vi "APC_PC_VariableMapping.vi"(3 "Index of array for 9056":i32[](array[numeric]), 4 "Index of array for 9049":i32[](array[numeric]), 5 "9056 IO":dbl[](array[numeric])=[0.0, 0.0, 0.0, 0.0, 0.0, 0.0, 0.0, 0.0, 0.0, 0.0, 0.0, 0.0, 0.0, 0.0, 0.0, 0.0, 0.0, 0.0, 0.0, 0.0, 0.0, 0.0, 0.0, 0.0, 0.0, 0.0, 0.0, 0.0, 0.0, 0.0, 0.0, 0.0, 0.0, 0.0, 0.0, 0.0, 0.0, 0.0, 0.0, 0.0, 0.0, 0.0, 0.0, 0.0, 0.0, 0.0, 0.0, 0.0, 0.0, 0.0], 6 "9049_CycleAveragedVariables":dbl[](array[numeric])=[5117258.0, 0.0, 0.0, 63.0, 1.0, 0.0, 0.0, 63.0, 94.902099609375, 1330.6719970703125, 0.00740314572500006, 0.028547040286386775, -1.6502519931731375e-05, 3.4809370619042162e-06, -1.939751072415059e-05, 0.04488519353144763, -3.310092996518957e-05, 1.9858346940817464e-05, -6.236978827880622e-06, 2.0827911733821188e-05, 9.443311193381779e-06, 0.006132818026759225, -2.7311908507416236e-05, 1.3270106306105403e-05, 0.028879043555142453, 0.028737060332811204, 0.028901641330023153, 22.045927206155966, 0.028741237014095793, 0.028786486597229075, 3.2774645046213114e-05, 1.6115711762159127e-05, 2.1821578936881718e-05, 0.03357141441039388, 2.0112356950239074e-05, 1.675670602532866e-05, 0.0006356573050482991, 0.0006466587796012424, 0.0007071076446904017, 289.1529637653157, 0.0006528559224250826, 0.0007237814910095489, 0.059188218510859716, 0.05131046864297262, 0.08300608203243602, 36736.18864406686, 0.06052347063369432, 0.0677338701327141, -28.066933770679075, -35.78734804893683, -36.11001435161502, -33.06495206371709, -31.40200617933432, -30.722872008289617, 18.300716235775724, 18.181513282367064, 13.746810443478878, 15.164170679724648, 24.37164065478366, 24.084193811561462, 44.362775965918274, 42.64924256286599, 48.52728616993939, 45.13534864860992, 44.56533514589826, 47.67972887407302, 539392.0, 539392.0]) -> (0 "Index 9056":i32[](array[numeric])=[-1, -1, -1, -1, -1, -1, -1, -1, -1, -1, -1, -1, -1, -1, -1, -1, -1, -1, -1, -1, -1, -1, -1, -1, -1, -1, -1, -1, -1, -1, -1, -1, -1, -1, -1, -1, -1, -1, -1, -1, -1, -1, -1, -1, -1, -1, -1, -1, -1, -1, -1, -1, -1, -1, -1, -1, -1, -1, -1, -1, -1, -1, -1, -1, -1, -1, -1, -1, -1, -1, -1, -1, -1, -1, -1, -1, -1, -1, -1, -1, -1, -1, -1, -1, -1, 2, 3, -1, -1, -1, 4, 5, 6, 7, 8, -1, 1, -1, -1, -1, -1, -1, -1, -1, -1, -1, -1, -1, -1, -1, -1, -1], 1 "Index 9049":i32[](array[numeric])=[-1, -1, -1, -1, -1, -1, -1, -1, -1, -1, -1, -1, -1, -1, -1, -1, -1, -1, -1, -1, -1, -1, -1, 18, 19, 20, 21, 22, 23, 30, 31, 32, 33, 34, 35, -1, -1, -1, -1, -1, -1, -1, -1, -1, -1, -1, -1, -1, -1, -1, -1, -1, -1, -1, 24, 25, 26, 27, 28, 29, -1, -1, -1, -1, -1, -1, -1, -1, -1, -1, -1, -1, -1, -1, -1, -1, -1, -1, -1, -1, -1, -1, -1, -1, -1, -1, -1, -1, -1, -1, -1, -1, -1, -1, -1, 9, -1, 66, 67, 36, 37, 38, 39, 40, 41, 54, 55, 56, 57, 58, 59, 8], 2 "Output cluster":T1 caption="Visualization cluster")   [LabVIEW 2020]
uses:
  controls/APC_VisualizationCluster_v2.ctl
  <vilib>/regexp/Match Regular Expression.xnode
  <vilib>/Utility/Data Type/NI_Data Type.lvlib
panel:
  out "Array":string[](array[string])
  out "Element 2":string[](array[string])=["Element not found", "Element not found", "Element not found", "Element not found", "Element not found", "Element not found", "Element not found", "Element not found", "Element not found", "Element not found", "Element not found", "Element not found", "Element not found", "Element not found", "Element not found", "Element not found", "Element not found", "Element not found", "Element not found", "Element not found", "Element not found", "Element not found", "Element not found", "IMEPn1", "IMEPn2", "IMEPn3", "IMEPn4", "IMEPn5", "IMEPn6", "IMEPstd1", "IMEPstd2", "IMEPstd3", "IMEPstd4", "IMEPstd5", "IMEPstd6", "Element not found", "Element not found", "Element not found", "Element not found", "Element not found", "Element not found", "Element not found", "Element not found", "Element not found", "Element not found", "Element not found", "Element not found", "Element not found", "Element not found", "Element not found", "Element not found", "Element not found", "Element not found", "Element not found", "MaxPcyl1", "MaxPcyl2", "MaxPcyl3", "MaxPcyl4", "MaxPcyl5", "MaxPcyl6", "Element not found", "Element not found", "Element not found", "Element not found", "Element not found", "Element not found", "Element not found", "Element not found", "Element not found", "Element not found", "Element not found", "Element not found", "Element not found", "Element not found", "Element not found", "Element not found", "Element not found", "Element not found", "Element not found", "Element not found", "Element not found", "Element not found", "Element not found", "Element not found", "Element not found", "Element not found", "Element not found", "Element not found", "Element not found", "Element not found", "Element not found", "Element not found", "Element not found", "Element not found", "Element not found", "EngineSpeed_rpm", "Element not found", "CylPresWarnings", "CylPresErrors", "MAPO1", "MAPO2", "MAPO3", "MAPO4", "MAPO5", "MAPO6", "CA50_1", "CA50_2", "CA50_3", "CA50_4", "CA50_5", "CA50_6", "SparkTiming"]
  out "x .or. y?":bool=TRUE
  out "Error Out 3":errorcluster
  in  "Ignore case":bool
  out "Element":string[](array[string])=["Element not found", "Element not found", "Element not found", "Element not found", "Element not found", "Element not found", "Element not found", "Element not found", "Element not found", "Element not found", "Element not found", "Element not found", "Element not found", "Element not found", "Element not found", "Element not found", "Element not found", "Element not found", "Element not found", "Element not found", "Element not found", "Element not found", "Element not found", "IMEPn1", "IMEPn2", "IMEPn3", "IMEPn4", "IMEPn5", "IMEPn6", "IMEPstd1", "IMEPstd2", "IMEPstd3", "IMEPstd4", "IMEPstd5", "IMEPstd6", "Element not found", "Element not found", "Element not found", "Element not found", "Element not found", "Element not found", "Element not found", "Element not found", "Element not found", "Element not found", "Element not found", "Element not found", "Element not found", "Element not found", "Element not found", "Element not found", "Element not found", "Element not found", "Element not found", "MaxPcyl1", "MaxPcyl2", "MaxPcyl3", "MaxPcyl4", "MaxPcyl5", "MaxPcyl6", "Element not found", "Element not found", "Element not found", "Element not found", "Element not found", "Element not found", "Element not found", "Element not found", "Element not found", "Element not found", "Element not found", "Element not found", "Element not found", "Element not found", "Element not found", "Element not found", "Element not found", "Element not found", "Element not found", "Element not found", "Element not found", "Element not found", "Element not found", "Element not found", "Element not found", "Element not found", "Element not found", "Element not found", "Element not found", "Element not found", "Element not found", "Element not found", "Element not found", "Element not found", "Element not found", "EngineSpeed_rpm", "Element not found", "CylPresWarnings", "CylPresErrors", "MAPO1", "MAPO2", "MAPO3", "MAPO4", "MAPO5", "MAPO6", "CA50_1", "CA50_2", "CA50_3", "CA50_4", "CA50_5", "CA50_6", "SparkTiming"]
  out "Error Out":errorcluster
  in  "Error In":errorcluster
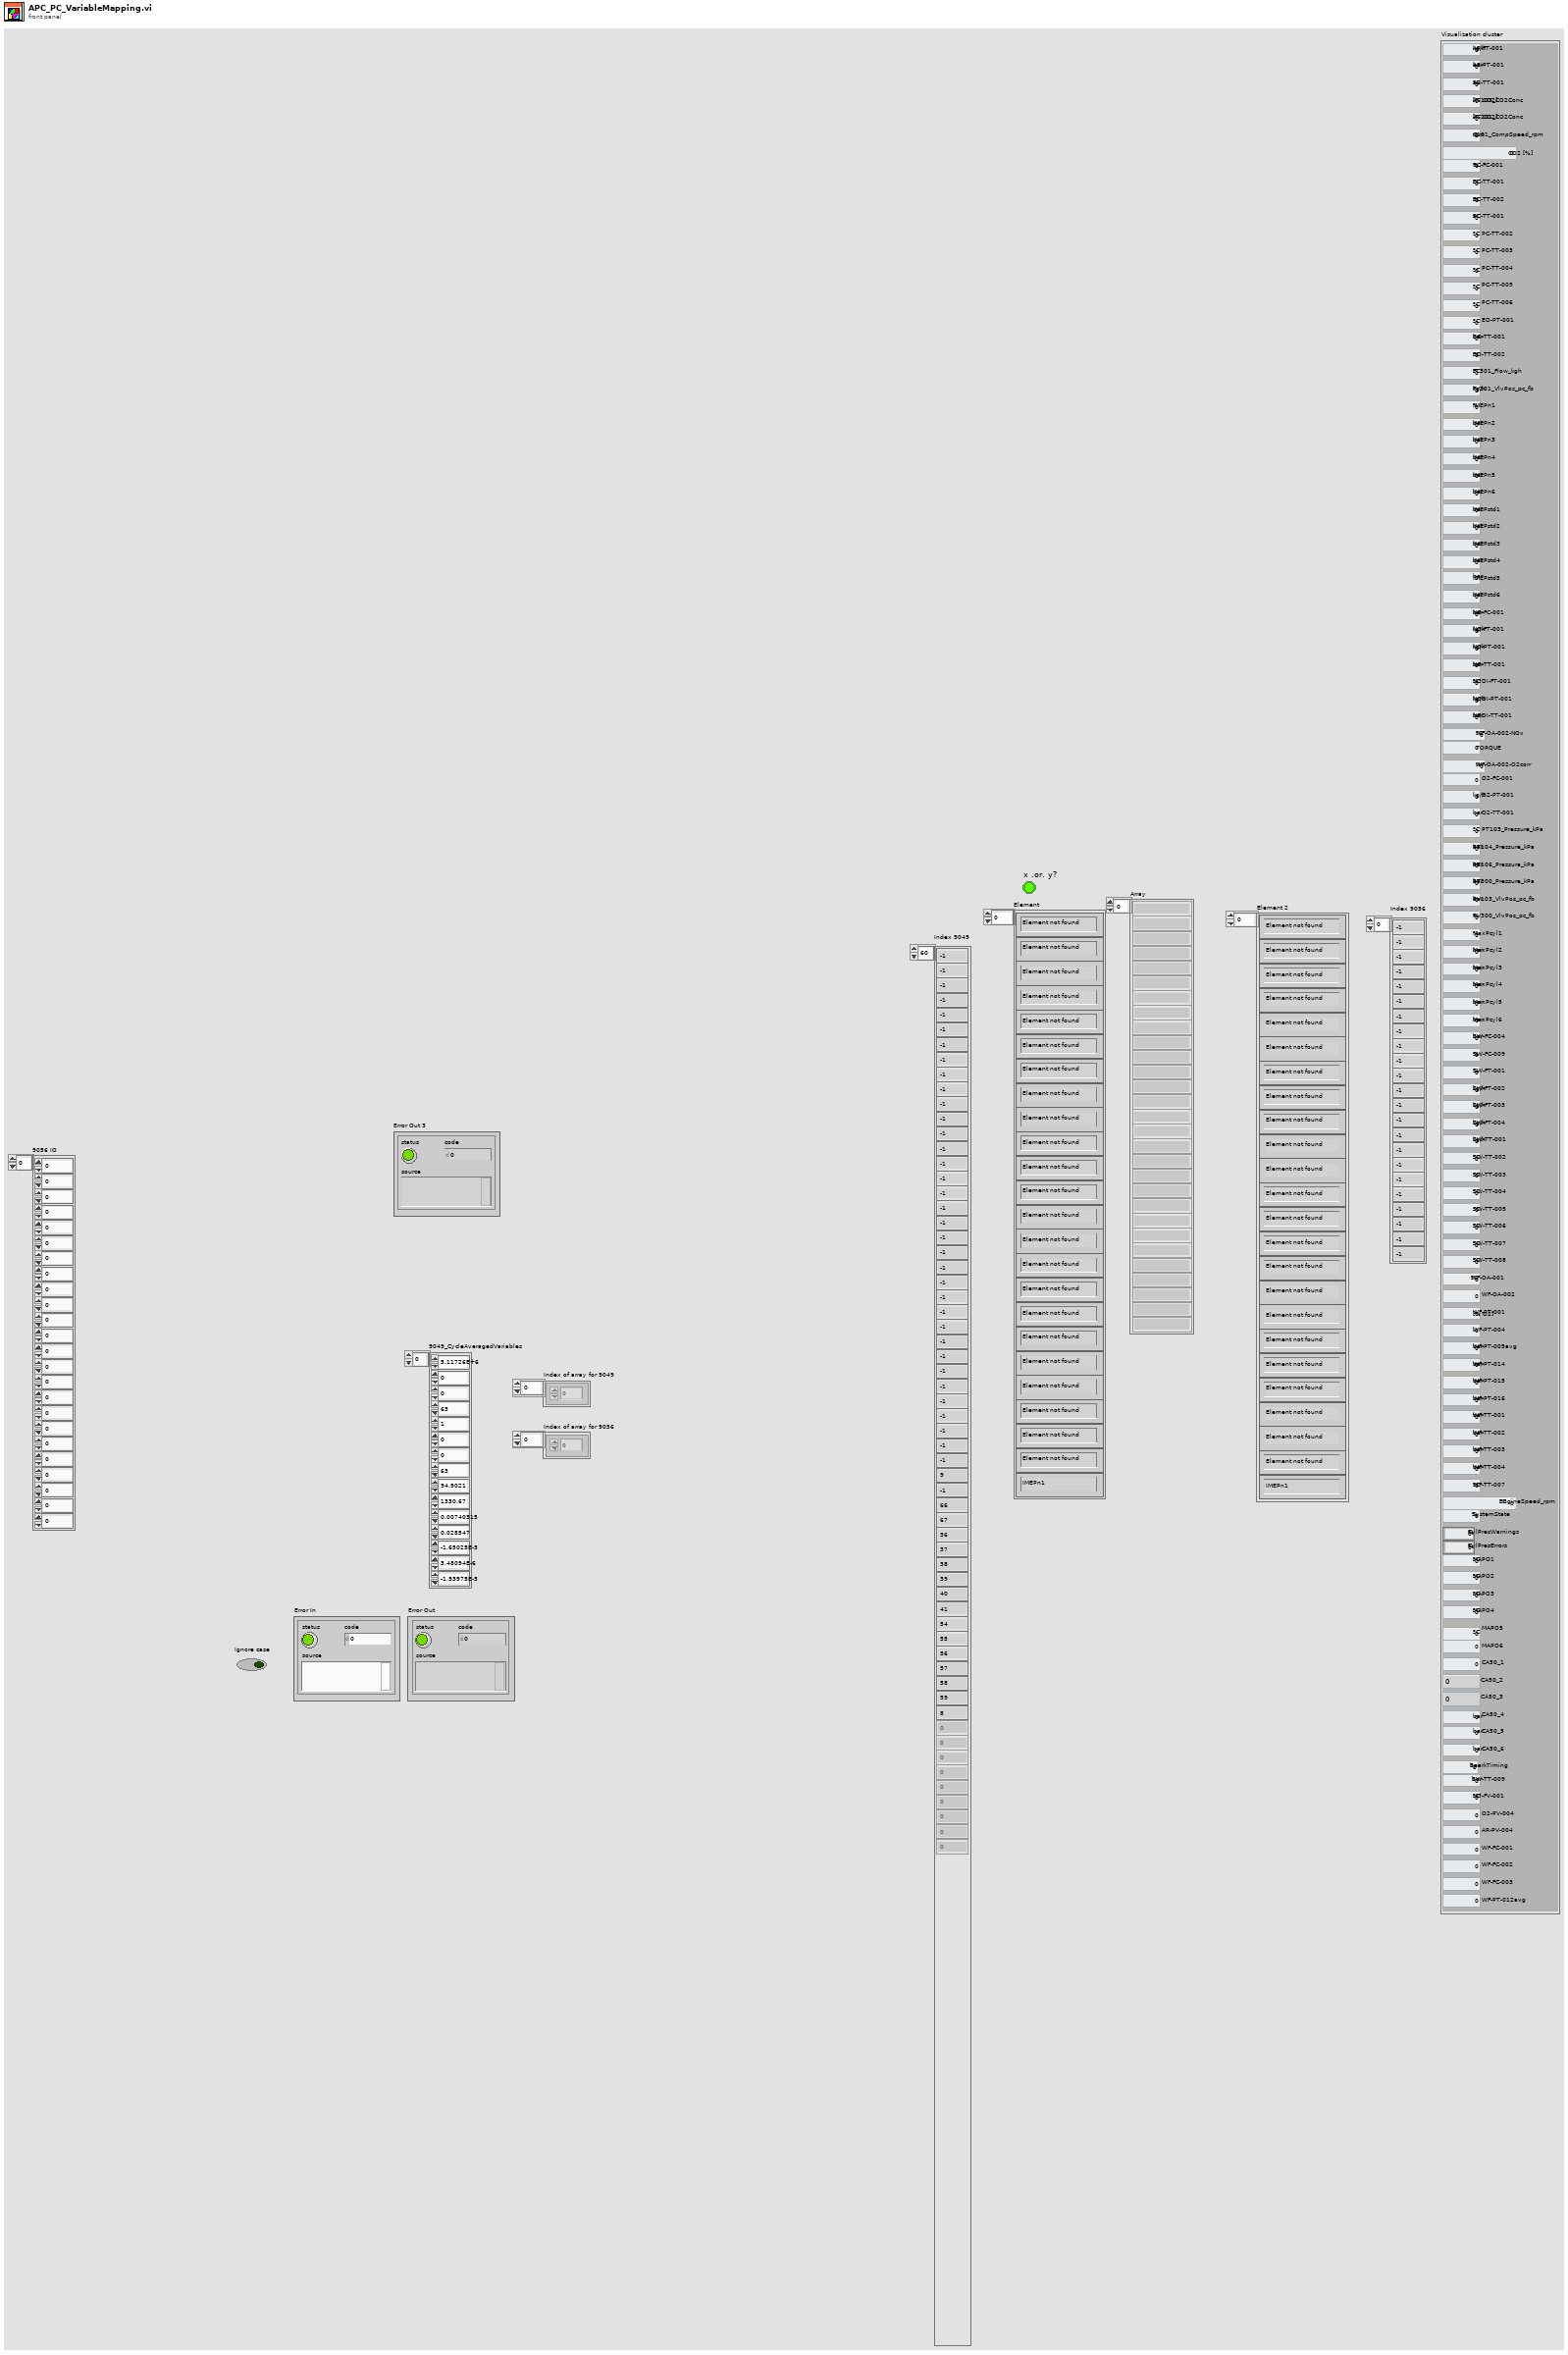
[diagram p1: front panel]
types:
  T1 = typedef "APC_VisualizationCluster_v2.ctl" = cluster{"AR-FT-001":dbl, "AR-PT-001":dbl, "AR-TT-001":dbl, "AT103_CO2Conc":dbl, "AT201_CO2Conc":dbl, "C101_CompSpeed_rpm":dbl, "CO2 [%]":dbl, "EC-FC-001":dbl, "EC-TT-001":dbl, "EC-TT-002":dbl, "PC-TT-001":dbl, "PC-TT-002":dbl, "PC-TT-003":dbl, "PC-TT-004":dbl, "PC-TT-005":dbl, "PC-TT-006":dbl, "EO-PT-001":dbl, "EO-TT-001":dbl, "EO-TT-002":dbl, "FT301_Flow_kgh":dbl, "FV301_VlvPos_pc_fb":dbl, "IMEPn1":dbl, "IMEPn2":dbl, "IMEPn3":dbl, "IMEPn4":dbl, "IMEPn5":dbl, "IMEPn6":dbl, "IMEPstd1":dbl, "IMEPstd2":dbl, "IMEPstd3":dbl, "IMEPstd4":dbl, "IMEPstd5":dbl, "IMEPstd6":dbl, "NG-FC-001":dbl, "NG-FT-001":dbl, "NG-PT-001":dbl, "NG-TT-001":dbl, "NGDI-FT-001":dbl, "NGDI-PT-001":dbl, "NGDI-TT-001":dbl, "WF-OA-002-NOx":dbl, "TORQUE":dbl, "WF-OA-002-O2corr":dbl, "O2-FC-001":dbl, "O2-PT-001":dbl, "O2-TT-001":dbl, "PT103_Pressure_kPa":dbl, "PT104_Pressure_kPa":dbl, "PT106_Pressure_kPa":dbl, "PT300_Pressure_kPa":dbl, "PV103_VlvPos_pc_fb":dbl, "PV300_VlvPos_pc_fb":dbl, "MaxPcyl1":dbl, "MaxPcyl2":dbl, "MaxPcyl3":dbl, "MaxPcyl4":dbl, "MaxPcyl5":dbl, "MaxPcyl6":dbl, "SW-FC-004":dbl, "SW-FC-009":dbl, "SW-FT-001":dbl, "SW-FT-002":dbl, "SW-FT-003":dbl, "SW-FT-004":dbl, "SW-TT-001":dbl, "SW-TT-002":dbl, "SW-TT-003":dbl, "SW-TT-004":dbl, "SW-TT-005":dbl, "SW-TT-006":dbl, "SW-TT-007":dbl, "SW-TT-008":dbl, "WF-OA-001":dbl, "WF-OA-002":dbl, "WF-PT-001":dbl, "WF-PT-004":dbl, "WF-PT-005avg":dbl, "WF-PT-014":dbl, "WF-PT-015":dbl, "WF-PT-016":dbl, "WF-TT-001":dbl, "WF-TT-002":dbl, "WF-TT-003":dbl, "WF-TT-004":dbl, "WF-TT-007":dbl, "EngineSpeed_rpm":dbl, "SystemState":dbl, "CylPresWarnings":dbl, "CylPresErrors":dbl, "MAPO1":dbl, "MAPO2":dbl, "MAPO3":dbl, "MAPO4":dbl, "MAPO5":dbl, "MAPO6":dbl, "CA50_1":dbl, "CA50_2":dbl, "CA50_3":dbl, "CA50_4":dbl, "CA50_5":dbl, "CA50_6":dbl, "SparkTiming":dbl, "SW-TT-009":dbl, "NG-FV-001":dbl, "O2-PV-004":dbl, "AR-PV-004":dbl, "WF-FC-001":dbl, "WF-FC-002":dbl, "WF-FC-003":dbl, "WF-PT-012avg":dbl}
  T2 = cluster{"[0]":dbl, "[1]":dbl, "[2]":dbl, "[3]":dbl, "[4]":dbl, "[5]":dbl, "[6]":dbl, "[7]":dbl, "[8]":dbl, "[9]":dbl, "[10]":dbl, "[11]":dbl, "[12]":dbl, "[13]":dbl, "[14]":dbl, "[15]":dbl, "[16]":dbl, "[17]":dbl, "[18]":dbl, "[19]":dbl, "[20]":dbl, "[21]":dbl, "[22]":dbl, "[23]":dbl, "[24]":dbl, "[25]":dbl, "[26]":dbl, "[27]":dbl, "[28]":dbl, "[29]":dbl, "[30]":dbl, "[31]":dbl, "[32]":dbl, "[33]":dbl, "[34]":dbl, "[35]":dbl, "[36]":dbl, "[37]":dbl, "[38]":dbl, "[39]":dbl, "[40]":dbl, "[41]":dbl, "[42]":dbl, "[43]":dbl, "[44]":dbl, "[45]":dbl, "[46]":dbl, "[47]":dbl, "[48]":dbl, "[49]":dbl, "[50]":dbl, "[51]":dbl, "[52]":dbl, "[53]":dbl, "[54]":dbl, "[55]":dbl, "[56]":dbl, "[57]":dbl, "[58]":dbl, "[59]":dbl, "[60]":dbl, "[61]":dbl, "[62]":dbl, "[63]":dbl, "[64]":dbl, "[65]":dbl, "[66]":dbl, "[67]":dbl, "[68]":dbl, "[69]":dbl, "[70]":dbl, "[71]":dbl, "[72]":dbl, "[73]":dbl, "[74]":dbl, "[75]":dbl, "[76]":dbl, "[77]":dbl, "[78]":dbl, "[79]":dbl, "[80]":dbl, "[81]":dbl, "[82]":dbl, "[83]":dbl, "[84]":dbl, "[85]":dbl, "[86]":dbl, "[87]":dbl, "[88]":dbl, "[89]":dbl, "[90]":dbl, "[91]":dbl, "[92]":dbl, "[93]":dbl, "[94]":dbl, "[95]":dbl, "[96]":dbl, "[97]":dbl, "[98]":dbl, "[99]":dbl, "[100]":dbl, "[101]":dbl, "[102]":dbl, "[103]":dbl, "[104]":dbl, "[105]":dbl, "[106]":dbl, "[107]":dbl, "[108]":dbl, "[109]":dbl, "[110]":dbl, "[111]":dbl, "[112]":dbl, "[113]":dbl, "[114]":dbl, "[115]":dbl, "[116]":dbl, "[117]":dbl, "[118]":dbl, "[119]":dbl, "[120]":dbl, "[121]":dbl, "[122]":dbl, "[123]":dbl, "[124]":dbl, "[125]":dbl, "[126]":dbl, "[127]":dbl, "[128]":dbl, "[129]":dbl, "[130]":dbl, "[131]":dbl, "[132]":dbl, "[133]":dbl, "[134]":dbl, "[135]":dbl, "[136]":dbl, "[137]":dbl, "[138]":dbl, "[139]":dbl, "[140]":dbl, "[141]":dbl, "[142]":dbl, "[143]":dbl, "[144]":dbl, "[145]":dbl, "[146]":dbl, "[147]":dbl, "[148]":dbl, "[149]":dbl, "[150]":dbl, "[151]":dbl, "[152]":dbl, "[153]":dbl, "[154]":dbl, "[155]":dbl, "[156]":dbl, "[157]":dbl, "[158]":dbl, "[159]":dbl, "[160]":dbl, "[161]":dbl, "[162]":dbl, "[163]":dbl, "[164]":dbl, "[165]":dbl, "[166]":dbl, "[167]":dbl, "[168]":dbl, "[169]":dbl, "[170]":dbl, "[171]":dbl, "[172]":dbl, "[173]":dbl, "[174]":dbl, "[175]":dbl, "[176]":dbl, "[177]":dbl, "[178]":dbl, "[179]":dbl, "[180]":dbl, "[181]":dbl, "[182]":dbl, "[183]":dbl, "[184]":dbl, "[185]":dbl, "[186]":dbl, "[187]":dbl, "[188]":dbl, "[189]":dbl, "[190]":dbl, "[191]":dbl, "[192]":dbl, "[193]":dbl, "[194]":dbl, "[195]":dbl, "[196]":dbl, "[197]":dbl, "[198]":dbl, "[199]":dbl, "[200]":dbl, "[201]":dbl, "[202]":dbl, "[203]":dbl, "[204]":dbl, "[205]":dbl, "[206]":dbl, "[207]":dbl, "[208]":dbl, "[209]":dbl, "[210]":dbl, "[211]":dbl, "[212]":dbl, "[213]":dbl, "[214]":dbl, "[215]":dbl, "[216]":dbl, "[217]":dbl, "[218]":dbl, "[219]":dbl, "[220]":dbl, "[221]":dbl, "[222]":dbl, "[223]":dbl, "[224]":dbl, "[225]":dbl, "[226]":dbl, "[227]":dbl, "[228]":dbl, "[229]":dbl, "[230]":dbl, "[231]":dbl, "[232]":dbl, "[233]":dbl, "[234]":dbl, "[235]":dbl, "[236]":dbl, "[237]":dbl, "[238]":dbl, "[239]":dbl, "[240]":dbl, "[241]":dbl, "[242]":dbl, "[243]":dbl, "[244]":dbl, "[245]":dbl, "[246]":dbl, "[247]":dbl, "[248]":dbl, "[249]":dbl, "[250]":dbl, "[251]":dbl, "[252]":dbl, "[253]":dbl, "[254]":dbl, "[255]":dbl}
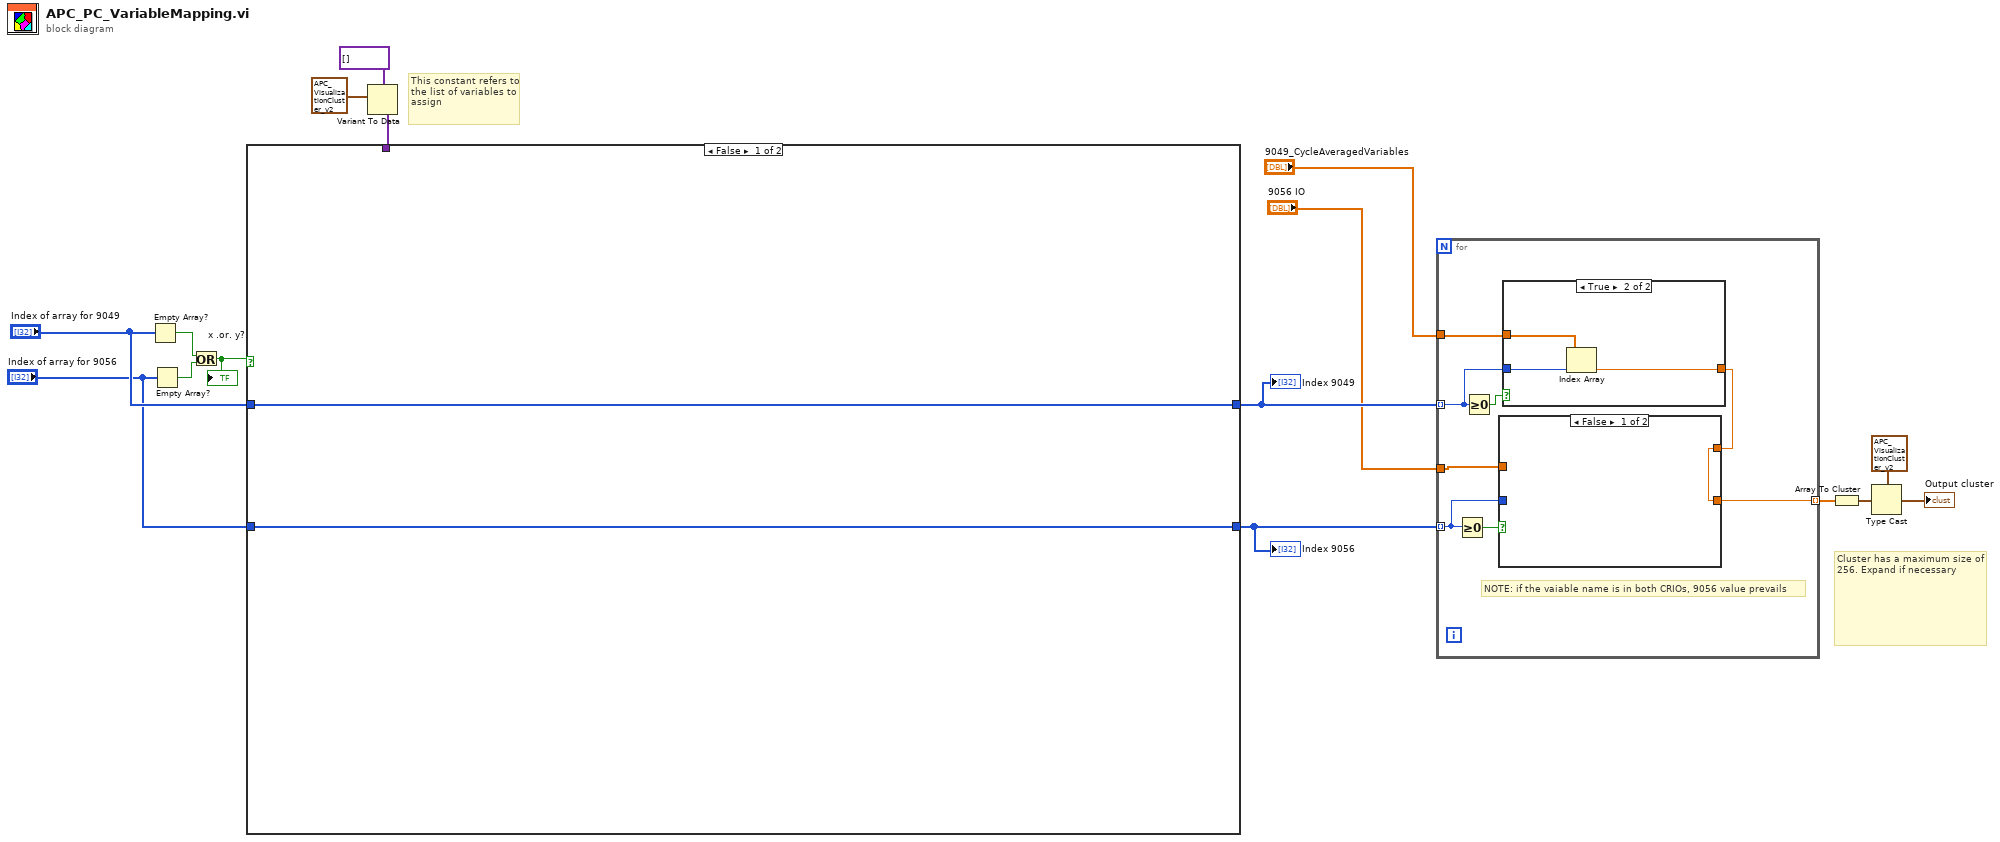
[diagram p0: block diagram]
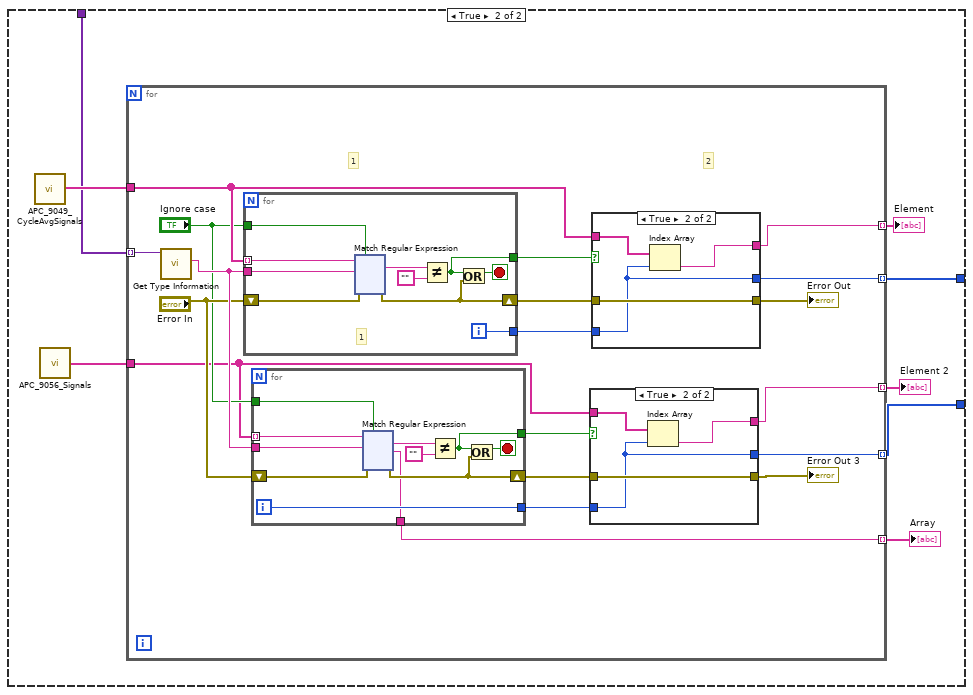
[diagram p2: hidden frame]
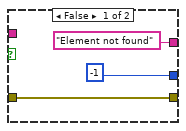
[diagram p3: hidden frame]
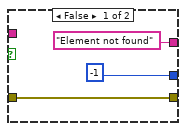
[diagram p4: hidden frame]
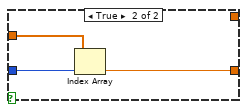
[diagram p5: hidden frame]
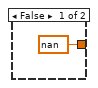
[diagram p6: hidden frame]
diagram:
  # "Cluster has a maximum size of 256. Expand if necessary"
  # "This constant refers to the list of variables to assign"
  n1 = Empty Array?(array="Index of array for 9049") -> (empty?=w9:bool)
  n2 = Empty Array?(array="Index of array for 9056") -> (empty?=w10:bool)
  n3 = Or(x=w9, y=w10) -> (x .or. y?=w8:bool)
  "x .or. y?" <- w8
  n4 = Variant To Data(type=variant[] [], Variant=T1 {"AR-FT-001"=0.0, "AR-PT-001"=0.0, "AR-TT-001"=0.0, "AT103_CO2Conc"=0.0, "AT201_CO2Conc"=0.0, "C101_CompSpeed_rpm"=0.0, "CO2 [%]"=0.0, "EC-FC-001"=0.0, "EC-TT-001"=0.0, "EC-TT-002"=0.0, "PC-TT-001"=0.0, "PC-TT-002"=0.0, "PC-TT-003"=0.0, "PC-TT-004"=0.0, "PC-TT-005"=0.0, "PC-TT-006"=0.0, "EO-PT-001"=0.0, "EO-TT-001"=0.0, "EO-TT-002"=0.0, "FT301_Flow_kgh"=0.0, "FV301_VlvPos_pc_fb"=0.0, "IMEPn1"=0.0, "IMEPn2"=0.0, "IMEPn3"=0.0, "IMEPn4"=0.0, "IMEPn5"=0.0, "IMEPn6"=0.0, "IMEPstd1"=0.0, "IMEPstd2"=0.0, "IMEPstd3"=0.0, "IMEPstd4"=0.0, "IMEPstd5"=0.0, "IMEPstd6"=0.0, "NG-FC-001"=0.0, "NG-FT-001"=0.0, "NG-PT-001"=0.0, "NG-TT-001"=0.0, "NGDI-FT-001"=0.0, "NGDI-PT-001"=0.0, "NGDI-TT-001"=0.0, "WF-OA-002-NOx"=0.0, "TORQUE"=0.0, "WF-OA-002-O2corr"=0.0, "O2-FC-001"=0.0, "O2-PT-001"=0.0, "O2-TT-001"=0.0, "PT103_Pressure_kPa"=0.0, "PT104_Pressure_kPa"=0.0, "PT106_Pressure_kPa"=0.0, "PT300_Pressure_kPa"=0.0, "PV103_VlvPos_pc_fb"=0.0, "PV300_VlvPos_pc_fb"=0.0, "MaxPcyl1"=0.0, "MaxPcyl2"=0.0, "MaxPcyl3"=0.0, "MaxPcyl4"=0.0, "MaxPcyl5"=0.0, "MaxPcyl6"=0.0, "SW-FC-004"=0.0, "SW-FC-009"=0.0, "SW-FT-001"=0.0, "SW-FT-002"=0.0, "SW-FT-003"=0.0, "SW-FT-004"=0.0, "SW-TT-001"=0.0, "SW-TT-002"=0.0, "SW-TT-003"=0.0, "SW-TT-004"=0.0, "SW-TT-005"=0.0, "SW-TT-006"=0.0, "SW-TT-007"=0.0, "SW-TT-008"=0.0, "WF-OA-001"=0.0, "WF-OA-002"=0.0, "WF-PT-001"=0.0, "WF-PT-004"=0.0, "WF-PT-005avg"=0.0, "WF-PT-014"=0.0, "WF-PT-015"=0.0, "WF-PT-016"=0.0, "WF-TT-001"=0.0, "WF-TT-002"=0.0, "WF-TT-003"=0.0, "WF-TT-004"=0.0, "WF-TT-007"=0.0, "EngineSpeed_rpm"=0.0, "SystemState"=0.0, "CylPresWarnings"=0.0, "CylPresErrors"=0.0, "MAPO1"=0.0, "MAPO2"=0.0, "MAPO3"=0.0, "MAPO4"=0.0, "MAPO5"=0.0, "MAPO6"=0.0, "CA50_1"=0.0, "CA50_2"=0.0, "CA50_3"=0.0, "CA50_4"=0.0, "CA50_5"=0.0, "CA50_6"=0.0, "SparkTiming"=0.0, "SW-TT-009"=0.0, "NG-FV-001"=0.0, "O2-PV-004"=0.0, "AR-PV-004"=0.0, "WF-FC-001"=0.0, "WF-FC-002"=0.0, "WF-FC-003"=0.0, "WF-PT-012avg"=0.0} ("Visualization cluster")) -> (data=w11:variant[])  [unwired: 1 in, 1 out]
  n5 = case shown="False" w8 {
    tunnel: "Index of array for 9049" -> [w18 _]
    tunnel: [w18 w26] -> w15
    tunnel: w11 -> [_ w24]
    tunnel: "Index of array for 9056" -> [w17 _]
    tunnel: [w17 w22] -> w6
    frame False {
    }
    frame True {
      n6 = call "APC_9049_CycleAvgSignals.vi"() -> ("CRIo9049_CycleAvgSignals"=w25:string[])  [unwired: 3 in]
      n7 = call "APC_9056_Signals.vi"() -> ("9056_raster"=w23:string[])  [unwired: 3 in, 2 out]
      n8 = for {
        tunnel: w25 -> [w41]
        tunnel: [w40] -> w26 mode=indexing
        tunnel: w24 -> [w39] mode=indexing
        tunnel: w23 -> [w32]
        tunnel: [w30] -> w22 mode=indexing
        tunnel: [w29] -> w21 mode=indexing
        tunnel: [w28] -> w20 mode=indexing
        tunnel: [w27] -> w19 mode=indexing
        # "1"
        # "2"
        # "1"
        n9 = call <vilib>:"Get Type Information.vi"("variant"=w39) -> ("name"=w38:string)  [unwired: 6 in, 4 out]
        n10 = for {
          tunnel: w41 -> [w191] mode=indexing
          tunnel: [w188] -> w44
          tunnel: w38 -> [w189]
          shift-right: [w182] -> w43
          shift-left: "Error In" -> [w183]
          tunnel: [w186] -> w45
          tunnel: "Ignore case" -> [w184]
          i -> [w188]
          stop <- w185 stop-if-true
          n11 = xnode "Match Regular Expression"("input string"=w191, "regular expression"=w189, "error in"=w183, "ignore case? (F)"=w184) -> ("whole match"=w190:string, "error out"=w182:errorcluster)  [unwired: 2 in, 3 out]
          n12 = Not Equal?(x=w190, y="") -> (x != y?=w186:bool)
          n13 = Or(x=w186, y=w182) -> (x .or. y?=w185:bool)
        }
        n14 = for {
          tunnel: w32 -> [w63] mode=indexing
          tunnel: [w60] -> w31
          tunnel: w38 -> [w61]
          shift-right: [w54] -> w34
          shift-left: "Error In" -> [w55]
          tunnel: [w58] -> w35
          tunnel: "Ignore case" -> [w56]
          tunnel: [w53] -> w27
          i -> [w60]
          stop <- w57 stop-if-true
          n15 = xnode "Match Regular Expression"("input string"=w63, "regular expression"=w61, "error in"=w55, "ignore case? (F)"=w56) -> ("whole match"=w62:string, "after match"=w53:string, "error out"=w54:errorcluster)  [unwired: 2 in, 2 out]
          n16 = Not Equal?(x=w62, y="") -> (x != y?=w58:bool)
          n17 = Or(x=w58, y=w54) -> (x .or. y?=w57:bool)
        }
        n18 = case shown="True" w35 {
          tunnel: w31 -> [_ w49]
          tunnel: w32 -> [_ w52]
          tunnel: ["Element not found" ("String") w51] -> w28
          tunnel: [-1 w49] -> w30
          tunnel: w34 -> [w46 w50]
          tunnel: [w46 w50] -> w33
          frame False {
          }
          frame True {
            n19 = Index Array(array=w52, index=w49) -> (element=w51:string)
          }
        }
        "Error Out 3" <- w33
        n20 = case shown="True" w45 {
          tunnel: w44 -> [_ w178]
          tunnel: w41 -> [_ w181]
          tunnel: ["Element not found" ("String") w180] -> w29
          tunnel: [-1 w178] -> w40
          tunnel: w43 -> [w175 w179]
          tunnel: [w175 w179] -> w42
          frame False {
          }
          frame True {
            n21 = Index Array(array=w181, index=w178) -> (element=w180:string)
          }
        }
        "Error Out" <- w42
      }
      "Element" <- w21
      "Element 2" <- w20
      "Array" <- w19
    }
  }
  "Index 9049" <- w15
  "Index 9056" <- w6
  n22 = for {
    tunnel: w15 -> [w307] mode=indexing
    tunnel: "9049_CycleAveragedVariables" -> [w310]
    tunnel: w6 -> [w306] mode=indexing
    tunnel: "9056 IO" -> [w309]
    tunnel: [w303] -> w2 mode=indexing
    # "NOTE: if the vaiable name is in both CRIOs, 9056 value prevails"
    n23 = Greater Or Equal To 0?(x=w306) -> (x >= 0?=w305:bool)
    n24 = Greater Or Equal To 0?(x=w307) -> (x >= 0?=w308:bool)
    n25 = case shown="True" w308 {
      tunnel: w310 -> [_ w318]
      tunnel: w307 -> [_ w317]
      tunnel: [nan ("millisecond timer value") w316] -> w304
      frame False {
      }
      frame True {
        n26 = Index Array(array=w318, index=w317) -> (element=w316:dbl)
      }
    }
    n27 = case shown="False" w305 {
      tunnel: w309 -> [_ w314]
      tunnel: w306 -> [_ w313]
      tunnel: [w311 w312] -> w303
      tunnel: w304 -> [w311 _]
      frame False {
      }
      frame True {
        n28 = Index Array(array=w314, index=w313) -> (element=w312:dbl)
      }
    }
  }
  n29 = Array To Cluster(array=w2) -> (cluster=w4:T2)
  n30 = Type Cast(type=T1 {"AR-FT-001"=0.0, "AR-PT-001"=0.0, "AR-TT-001"=0.0, "AT103_CO2Conc"=0.0, "AT201_CO2Conc"=0.0, "C101_CompSpeed_rpm"=0.0, "CO2 [%]"=0.0, "EC-FC-001"=0.0, "EC-TT-001"=0.0, "EC-TT-002"=0.0, "PC-TT-001"=0.0, "PC-TT-002"=0.0, "PC-TT-003"=0.0, "PC-TT-004"=0.0, "PC-TT-005"=0.0, "PC-TT-006"=0.0, "EO-PT-001"=0.0, "EO-TT-001"=0.0, "EO-TT-002"=0.0, "FT301_Flow_kgh"=0.0, "FV301_VlvPos_pc_fb"=0.0, "IMEPn1"=0.0, "IMEPn2"=0.0, "IMEPn3"=0.0, "IMEPn4"=0.0, "IMEPn5"=0.0, "IMEPn6"=0.0, "IMEPstd1"=0.0, "IMEPstd2"=0.0, "IMEPstd3"=0.0, "IMEPstd4"=0.0, "IMEPstd5"=0.0, "IMEPstd6"=0.0, "NG-FC-001"=0.0, "NG-FT-001"=0.0, "NG-PT-001"=0.0, "NG-TT-001"=0.0, "NGDI-FT-001"=0.0, "NGDI-PT-001"=0.0, "NGDI-TT-001"=0.0, "WF-OA-002-NOx"=0.0, "TORQUE"=0.0, "WF-OA-002-O2corr"=0.0, "O2-FC-001"=0.0, "O2-PT-001"=0.0, "O2-TT-001"=0.0, "PT103_Pressure_kPa"=0.0, "PT104_Pressure_kPa"=0.0, "PT106_Pressure_kPa"=0.0, "PT300_Pressure_kPa"=0.0, "PV103_VlvPos_pc_fb"=0.0, "PV300_VlvPos_pc_fb"=0.0, "MaxPcyl1"=0.0, "MaxPcyl2"=0.0, "MaxPcyl3"=0.0, "MaxPcyl4"=0.0, "MaxPcyl5"=0.0, "MaxPcyl6"=0.0, "SW-FC-004"=0.0, "SW-FC-009"=0.0, "SW-FT-001"=0.0, "SW-FT-002"=0.0, "SW-FT-003"=0.0, "SW-FT-004"=0.0, "SW-TT-001"=0.0, "SW-TT-002"=0.0, "SW-TT-003"=0.0, "SW-TT-004"=0.0, "SW-TT-005"=0.0, "SW-TT-006"=0.0, "SW-TT-007"=0.0, "SW-TT-008"=0.0, "WF-OA-001"=0.0, "WF-OA-002"=0.0, "WF-PT-001"=0.0, "WF-PT-004"=0.0, "WF-PT-005avg"=0.0, "WF-PT-014"=0.0, "WF-PT-015"=0.0, "WF-PT-016"=0.0, "WF-TT-001"=0.0, "WF-TT-002"=0.0, "WF-TT-003"=0.0, "WF-TT-004"=0.0, "WF-TT-007"=0.0, "EngineSpeed_rpm"=0.0, "SystemState"=0.0, "CylPresWarnings"=0.0, "CylPresErrors"=0.0, "MAPO1"=0.0, "MAPO2"=0.0, "MAPO3"=0.0, "MAPO4"=0.0, "MAPO5"=0.0, "MAPO6"=0.0, "CA50_1"=0.0, "CA50_2"=0.0, "CA50_3"=0.0, "CA50_4"=0.0, "CA50_5"=0.0, "CA50_6"=0.0, "SparkTiming"=0.0, "SW-TT-009"=0.0, "NG-FV-001"=0.0, "O2-PV-004"=0.0, "AR-PV-004"=0.0, "WF-FC-001"=0.0, "WF-FC-002"=0.0, "WF-FC-003"=0.0, "WF-PT-012avg"=0.0} ("Visualization cluster"), x=w4) -> (*(type *) &x=→"Output cluster":T1)
